vi "Refname to String (Huskie Board).vi"(1 "Enum":T1) -> (0 "resulting string":string)   [LabVIEW 2016, in "Huskie Swerve.lvlib"]
uses:
  Huskie Swerve.lvlib
  Huskie Board.ctl
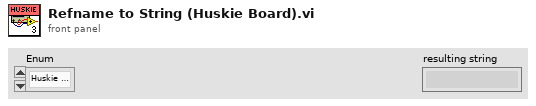
[diagram p1: front panel]
types:
  T1 = typedef "Huskie Swerve.lvlib/Huskie Board.ctl" = enum16{"Huskie Board", "Log Queue", ""}
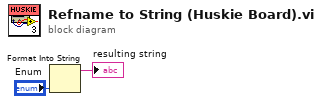
[diagram p0: block diagram]
diagram:
  n1 = Format Into String("Enum") -> (resulting string=→"resulting string":string)  [unwired: 3 in, 1 out]
